vi "ReSizeArray.vi"(8 "1D":dbl[](array[numeric]), 11 "2D":dbl[][](array[numeric])) -> (0 "2D":dbl[][](array[numeric]), 3 "1D":dbl[](array[numeric]))   [LabVIEW 2023]
panel:
  # "2D to"
  # "Взима само 1-я ред от 2D масива"
  # "1D to"
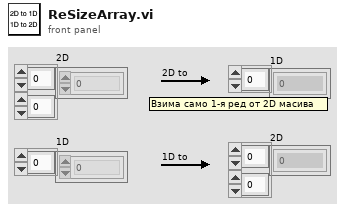
[diagram p1: front panel]
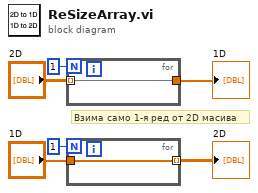
[diagram p0: block diagram]
diagram:
  # "Взима само 1-я ред от 2D масива"
  n1 = for {
    N: 1 -> [_]
    tunnel: "2D" -> [w7] mode=indexing
    tunnel: [w7] -> w5
  }
  "1D" <- w5
  n2 = for {
    N: 1 -> [_]
    tunnel: "1D" -> [w8]
    tunnel: [w8] -> w3 mode=indexing
  }
  "2D" <- w3
